vi "Convert Channel Values to Sine Generate Settings.vi"(9 "Length":i32, 10 "Index":i32, 11 "Channel Values in":dbl[](array[numeric])) -> (2 "Sine Generate Settings":T1, 3 "Channel Values out":dbl[](array[numeric]))   [LabVIEW 2018, in "FPGA Addon Engine.lvlib"]
uses:
  FPGA Addon Engine.lvlib
  Submodules/Source/Types/Sine.Generate.Settings.ctl
  Submodules/Source/Speciality FPGA IO.lvlib
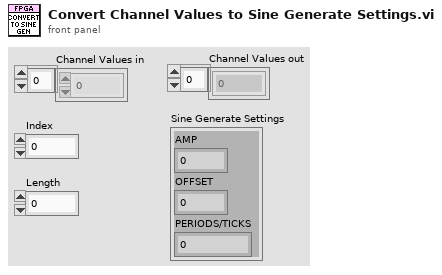
[diagram p1: front panel]
types:
  T1 = typedef "Speciality FPGA IO.lvlib/Sine.Generate.Settings.ctl" = cluster{"AMP":fxp<+/-,32,8>, "OFFSET":fxp<+/-,32,8>, "PERIODS/TICKS":fxp<+,32,0>}
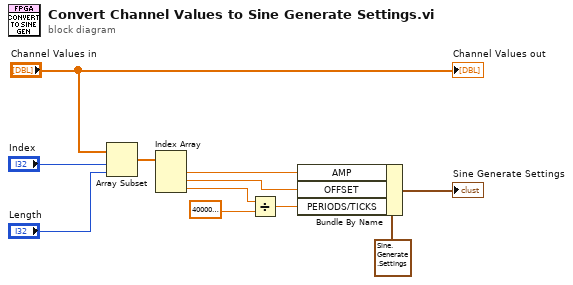
[diagram p0: block diagram]
diagram:
  n1 = Array Subset(array="Channel Values in", index="Index", length="Length") -> (w1:dbl[])
  n2 = Index Array(array=w1) -> (element #1=w5:dbl, element #2=w4:dbl, element #3=w3:dbl)  [unwired: 3 in]
  n3 = Divide(x=w3, y=sgl 40000000.0) -> (x/y=w6:dbl)
  n4 = Bundle By Name(cluster=T1 {"AMP"=0.0, "OFFSET"=0.0, "PERIODS/TICKS"=0.0} ("Settings"), "AMP"=w5, "OFFSET"=w4, "PERIODS/TICKS"=w6) -> (→"Sine Generate Settings":T1)
  "Channel Values out" <- "Channel Values in"
